vi "Fixup.vi"(5 "Format empty string as null":bool, 6 "Pretty Print Levels":i32, 7 "Alphabetically Sort Objects":bool, 8 "error in (no error)":errorcluster, 10 "Offset":i32, 11 "JSON":string) -> (0 "error out":errorcluster, 1 "Offset past":i32 caption="Offset past Value", 2 "Rest of Input String":string, 3 "<JSON>":string caption="<JSON>First JSON Value")   [LabVIEW 2017, in "JSONtext.lvlib"]
doc: "Reformat a JSON Value, either packed with all unneeded whitespace removed, or \"pretty printed\" with extra whitespace and new lines to make the JSON more human readable. This will also serve to validate the JSON.\n\n\"Pretty Print Levels\" is the number of deeper levels at which to apply pretty print. Use a high number to apply at all levels, and use zero to indicate no pretty print."
uses:
  JSONtext.lvlib
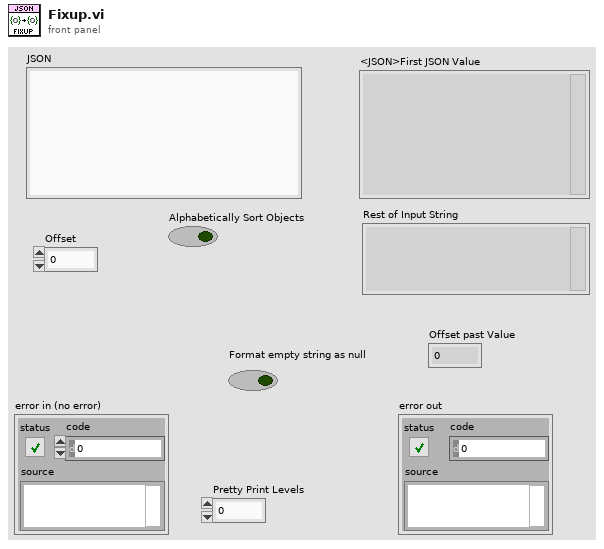
[diagram p1: front panel]
types:
  T1 = typedef "JSONtext.lvlib/Parsing State.ctl" = enum16{"Parser Error", "Object", "Array", "String", "Number/Other", "Leading Whitespace", "Object end", "Array end", "Value end"}
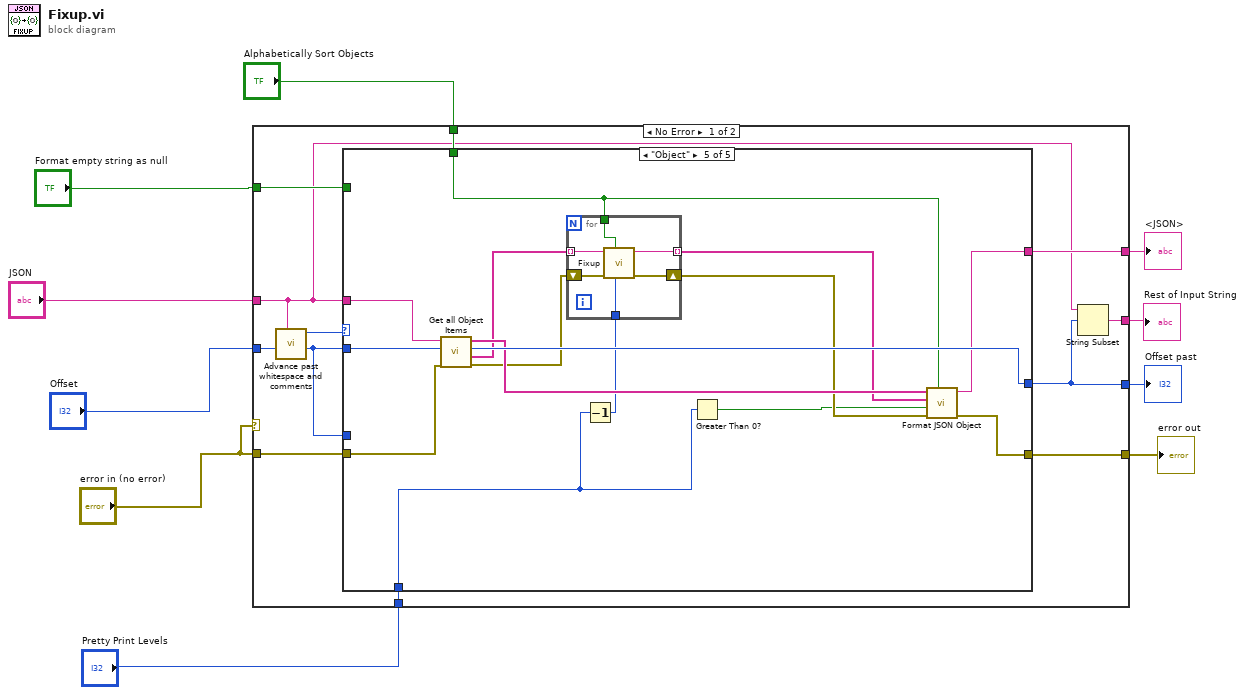
[diagram p0: block diagram]
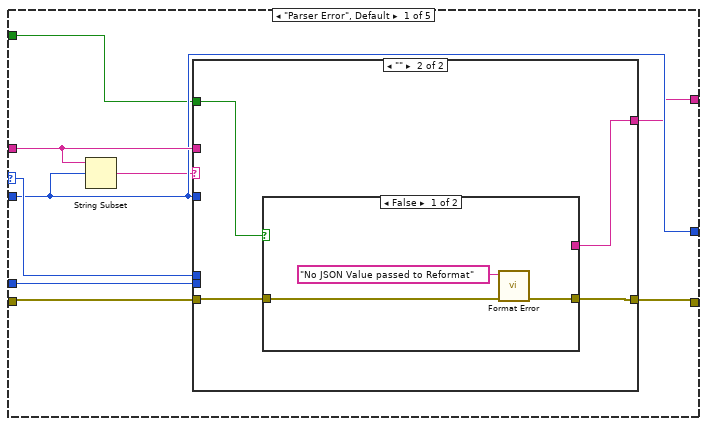
[diagram p2: hidden frame]
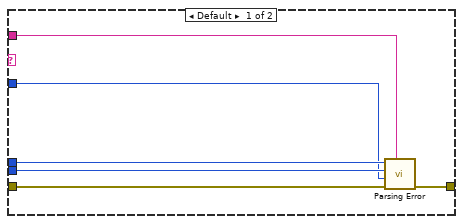
[diagram p3: hidden frame]
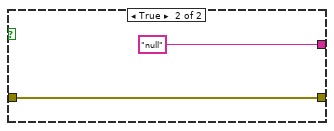
[diagram p4: hidden frame]
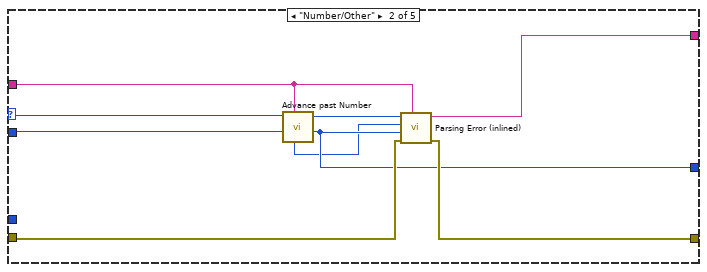
[diagram p5: hidden frame]
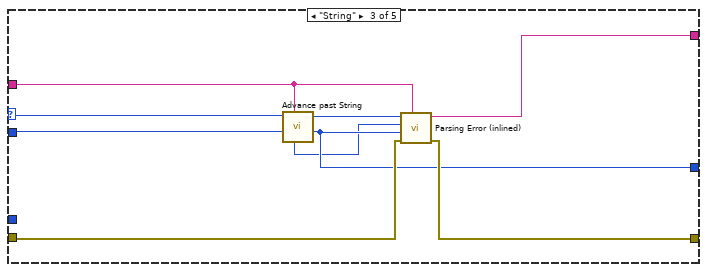
[diagram p6: hidden frame]
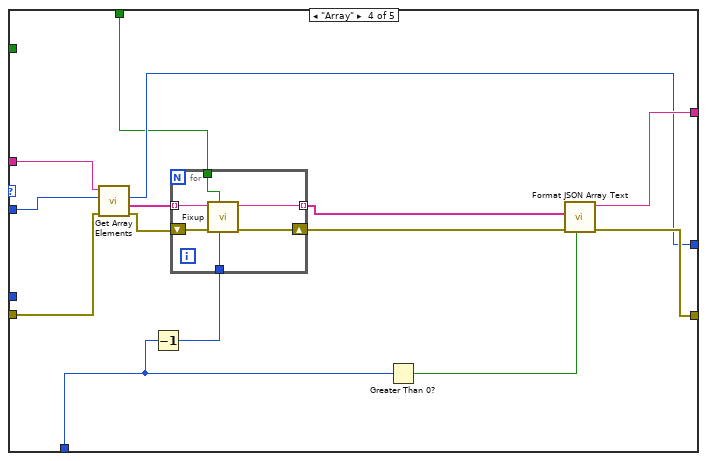
[diagram p7: hidden frame]
diagram:
  n1 = case shown="No Error" "error in (no error)" {
    tunnel: "JSON" -> [w11 w107]
    tunnel: "Offset" -> [w21 w108]
    tunnel: [w20 w106] -> w8
    tunnel: "error in (no error)" -> [w19 w106]
    tunnel: "Pretty Print Levels" -> [w17 _]
    tunnel: [w16 _] -> w6
    tunnel: [w15 w108] -> w5
    tunnel: [w14 w107] -> w4
    tunnel: "Alphabetically Sort Objects" -> [w13 _]
    tunnel: "Format empty string as null" -> [w12 _]
    frame No Error {
      n2 = call "Advance past whitespace and comments.vi"("JSON"=w11, "Offset"=w21) -> ("Offset of first non-whitespace"=w18:i32, "Parser State"=w22:T1)  [unwired: 8 in]
      n3 = case shown="\"Object\"" w22 {
        selector: w22 -> [w29 w55 w64 _ _]
        tunnel: w11 -> [w27 w48 w57 w78 w96]
        tunnel: w18 -> [w26 w54 w63 w77 w99]
        tunnel: [w26 w51 w60 w71 w98] -> w15
        tunnel: [w24 w47 w56 w75 w95] -> w16
        tunnel: [w31 w52 w61 w73 w90] -> w20
        tunnel: w19 -> [w30 w53 w62 w72 w89]
        tunnel: w18 -> [w28 _ _ _ _]
        tunnel: w17 -> [_ _ _ w68 w87]
        tunnel: w13 -> [_ _ _ w65 w85]
        tunnel: w12 -> [w23 _ _ _ _]
        frame "Parser Error", Default {
          n4 = String Subset(string=w27, offset (0)=w26) -> (substring=w25:string)  [unwired: 1 in]
          n5 = case shown="\"\"" w25 {
            tunnel: [w37 w40] -> w31
            tunnel: w30 -> [w36 w41]
            tunnel: w29 -> [w35 _]
            tunnel: w28 -> [w34 _]
            tunnel: w27 -> [w33 _]
            tunnel: w26 -> [w32 _]
            tunnel: [_ w38] -> w24
            tunnel: w23 -> [_ w39]
            frame Default {
              n6 = call "Parsing Error.vi"("JSON"=w33, "error in (no error)"=w36, "Offset past match"=w32, "Value start"=w34, "State"=w35) -> ("error out"=w37:errorcluster)  [unwired: 6 in]
            }
            frame "" {
              n7 = case shown="False" w39 {
                tunnel: w41 -> [w44 w46]
                tunnel: [w43 w46] -> w40
                tunnel: [_ "null"] -> w38
                frame False {
                  n8 = call "Format Error.vi"("error in (no error)"=w44, "error message"="No JSON Value passed to Reformat") -> ("error out"=w43:errorcluster)  [unwired: 9 in]
                }
                frame True {
                }
              }
            }
          }
        }
        frame "Number/Other" {
          n9 = call "Advance past Number.vi"("JSON"=w48, "Offset (0)"=w54, "Parser State in"=w55) -> ("Offset past match"=w51:i32, "Parser State"=w49:T1, "Value start out"=w50:i32)  [unwired: 5 in, 1 out]
          n10 = call "Parsing Error (inlined).vi"("JSON"=w48, "error in (no error)"=w53, "Offset past match"=w51, "Value start"=w50, "State"=w49) -> ("error out"=w52:errorcluster, "Value (if no error)"=w47:string)  [unwired: 5 in]
        }
        frame "String" {
          n11 = call "Advance past String.vi"("JSON"=w57, "Offset"=w63, "State in"=w64) -> ("Offset past match"=w60:i32, "State"=w58:T1, "Value start out"=w59:i32)  [unwired: 6 in]
          n12 = call "Parsing Error (inlined).vi"("JSON"=w57, "error in (no error)"=w62, "Offset past match"=w60, "Value start"=w59, "State"=w58) -> ("error out"=w61:errorcluster, "Value (if no error)"=w56:string)  [unwired: 5 in]
        }
        frame "Array" {
          n13 = call "Get Array Elements.vi"("error in (no error)"=w72, "Offset"=w77, "JSON"=w78) -> ("error out"=w74:errorcluster, "<JSON>"=w76:string[], "Offset past"=w71:i32)  [unwired: 6 in]
          n14 = Decrement(x=w68) -> (x-1=w67:i32)
          n15 = for {
            tunnel: w76 -> [w84] mode=indexing
            tunnel: [w83] -> w70 mode=indexing
            shift-right: [w81] -> w69
            shift-left: w74 -> [w82]
            tunnel: w67 -> [w80]
            tunnel: w65 -> [w79]
            n16 = call "Fixup.vi"("Pretty Print Levels"=w80, "Alphabetically Sort Objects"=w79, "error in (no error)"=w82, "JSON"=w84) -> ("error out"=w81:errorcluster, "<JSON>"=w83:string)  [unwired: 4 in, 2 out]
          }
          n17 = Greater Than 0?(x=w68) -> (x > 0?=w66:bool)
          n18 = call "Format JSON Array Text.vi"("Pretty Print?"=w66, "error in (no error)"=w69, "Array of JSON Text"=w70) -> ("error out"=w73:errorcluster, "<JSON>"=w75:string)  [unwired: 7 in]
        }
        frame "Object" {
          n19 = call "Get all Object Items.vi"("error in (no error)"=w89, "Offset"=w99, "JSON"=w96) -> ("error out"=w92:errorcluster, "<JSON>"=w94:string[], "Offset past"=w98:i32, "Item Names"=w97:string[])  [unwired: 5 in]
          n20 = Decrement(x=w87) -> (x-1=w86:i32)
          n21 = for {
            tunnel: w94 -> [w105] mode=indexing
            tunnel: [w104] -> w93 mode=indexing
            shift-right: [w102] -> w91
            shift-left: w92 -> [w103]
            tunnel: w86 -> [w101]
            tunnel: w85 -> [w100]
            n22 = call "Fixup.vi"("Pretty Print Levels"=w101, "Alphabetically Sort Objects"=w100, "error in (no error)"=w103, "JSON"=w105) -> ("error out"=w102:errorcluster, "<JSON>"=w104:string)  [unwired: 4 in, 2 out]
          }
          n23 = Greater Than 0?(x=w87) -> (x > 0?=w88:bool)
          n24 = call "Format JSON Object.vi"("Alphabetical Sort"=w85, "error in (no error)"=w91, "Pretty Print?"=w88, "JSON elements"=w93, "Names"=w97) -> ("error out"=w90:errorcluster, "JSON Object Text out"=w95:string)  [unwired: 5 in]
        }
      }
      n25 = String Subset(string=w11, offset (0)=w15) -> (substring=w14:string)  [unwired: 1 in]
    }
    frame Error {
    }
  }
  "Offset past" <- w5
  "<JSON>" <- w6
  "error out" <- w8
  "Rest of Input String" <- w4
